vi "ShotSelector.vi"(11 "Buttons":bool[](array[boolean])=[FALSE, FALSE, FALSE, FALSE, FALSE, FALSE, FALSE, FALSE, FALSE, FALSE, FALSE, FALSE, FALSE, FALSE, FALSE, FALSE, FALSE, FALSE, FALSE, FALSE, FALSE, FALSE, FALSE, FALSE, FALSE, FALSE, FALSE, FALSE, FALSE, FALSE, FALSE, FALSE]) -> ()   [LabVIEW 2015]
uses:
  Utilities/MotorPositionGlobals.vi
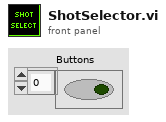
[diagram p1: front panel]
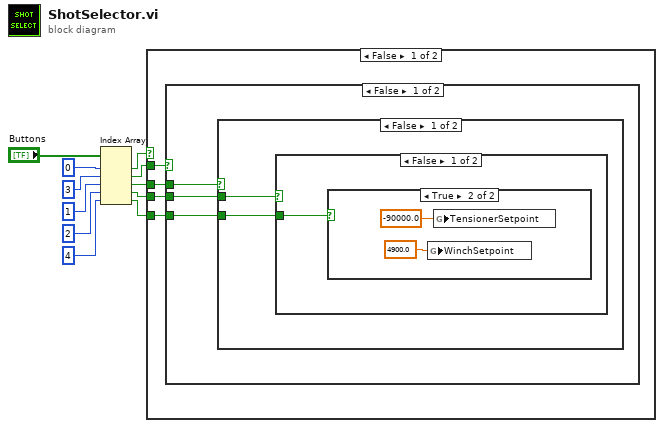
[diagram p0: block diagram]
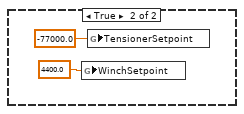
[diagram p3: hidden frame]
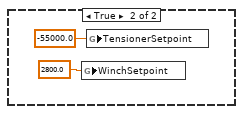
[diagram p4: hidden frame]
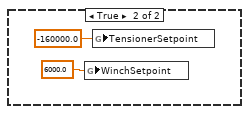
[diagram p5: hidden frame]
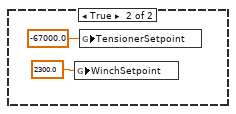
[diagram p6: hidden frame]
diagram:
  n1 = Index Array(array="Buttons", index #1=0 ("index"), index #2=3 ("index"), index #3=1 ("index"), index #4=2 ("index"), index #5=4 ("index")) -> (element #1=w7:bool, element #2=w6:bool, element #3=w5:bool, element #4=w3:bool, element #5=w1:bool)
  n2 = case shown="False" w7 {
    tunnel: w6 -> [w15 _]
    tunnel: w5 -> [w14 _]
    tunnel: w3 -> [w13 _]
    tunnel: w1 -> [w12 _]
    frame False {
      n3 = case shown="False" w15 {
        tunnel: w14 -> [w18 _]
        tunnel: w13 -> [w17 _]
        tunnel: w12 -> [w16 _]
        frame False {
          n4 = case shown="False" w18 {
            tunnel: w17 -> [w20 _]
            tunnel: w16 -> [w19 _]
            frame False {
              n5 = case shown="False" w20 {
                tunnel: w19 -> [w21 _]
                frame False {
                  n6 = case shown="True" w21 {
                    frame False {
                    }
                    frame True {
                      n7 = global write "MotorPositionGlobals.vi" "WinchSetpoint"(4900.0 ("WinchSetpoint")) -> ()
                      n8 = global write "MotorPositionGlobals.vi" "TensionerSetpoint"(-90000.0 ("TensionerSetpoint")) -> ()
                    }
                  }
                }
                frame True {
                  n9 = global write "MotorPositionGlobals.vi" "WinchSetpoint"(4400.0 ("WinchSetpoint")) -> ()
                  n10 = global write "MotorPositionGlobals.vi" "TensionerSetpoint"(-77000.0 ("TensionerSetpoint")) -> ()
                }
              }
            }
            frame True {
              n11 = global write "MotorPositionGlobals.vi" "WinchSetpoint"(2800.0 ("WinchSetpoint")) -> ()
              n12 = global write "MotorPositionGlobals.vi" "TensionerSetpoint"(-55000.0 ("TensionerSetpoint")) -> ()
            }
          }
        }
        frame True {
          n13 = global write "MotorPositionGlobals.vi" "WinchSetpoint"(6000.0 ("WinchSetpoint")) -> ()
          n14 = global write "MotorPositionGlobals.vi" "TensionerSetpoint"(-160000.0 ("TensionerSetpoint")) -> ()
        }
      }
    }
    frame True {
      n15 = global write "MotorPositionGlobals.vi" "WinchSetpoint"(2300.0 ("WinchSetpoint 2")) -> ()
      n16 = global write "MotorPositionGlobals.vi" "TensionerSetpoint"(-67000.0 ("TensionerSetpoint 2")) -> ()
    }
  }
